vi "Send string wait for return.vi"(0 "VISA resource":refnum<visa-resource-name>, 7 "Command string":string, 9 "Reply expected":bool, 11 "error IO":errorcluster) -> (4 "VISA resource out":refnum<visa-resource-name>, 8 "Reply string":string, 10 "Transmitted":string, 14 "Received Reply":bool, 15 "error out":errorcluster)   [LabVIEW 2011]
doc: "Send a text string to PCP og vent på resultatet om dette er valgt"
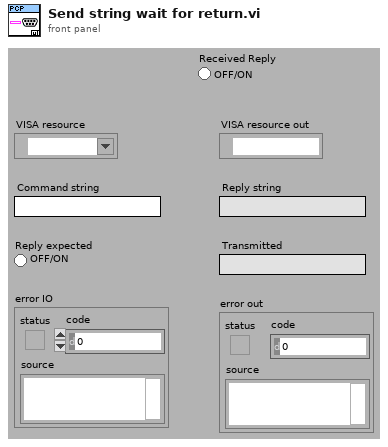
[diagram p1: front panel]
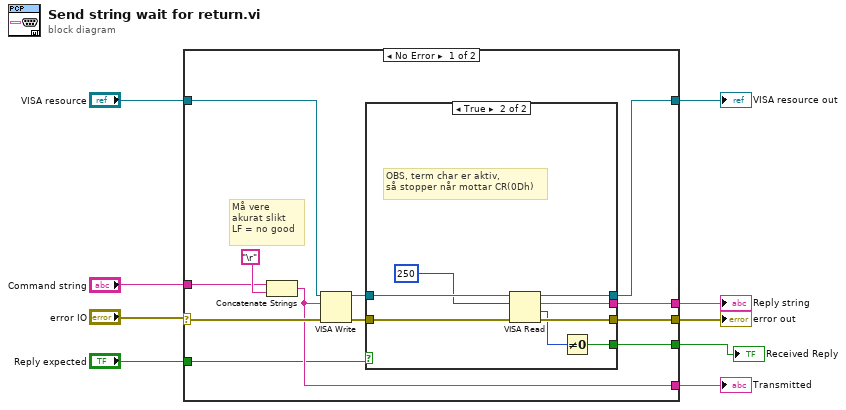
[diagram p0: block diagram]
diagram:
  n1 = case shown="No Error" "error IO" {
    selector: "error IO" -> [w21 w32]
    tunnel: [w17 w33] -> w2
    tunnel: "VISA resource" -> [w20 w33]
    tunnel: [w16 w32] -> w4
    tunnel: [w14 _] -> w5
    tunnel: [w13 _] -> w6
    tunnel: "Command string" -> [w12 _]
    tunnel: "Reply expected" -> [w11 _]
    tunnel: [w10 _] -> w1
    frame No Error {
      # "Må vere \nakurat slikt\nLF = no good"
      n2 = Concatenate Strings(w12, "\r") -> (w14:string)
      n3 = VISA Write(VISA resource name=w20, write buffer=w14, error in (no error)=w21) -> (VISA resource name out=w18:refnum<visa-resource-name>, error out=w19:errorcluster)  [unwired: 1 out]
      n4 = case shown="True" w11 {
        tunnel: w19 -> [w22 w31]
        tunnel: w18 -> [w23 w30]
        tunnel: [w23 w29] -> w17
        tunnel: [w22 w27] -> w16
        tunnel: [_ w26] -> w13
        tunnel: [_ w24] -> w10
        frame False {
          # "Ingen retur forventet"
        }
        frame True {
          # "OBS, term char er aktiv,\nså stopper når mottar CR(0Dh)"
          n5 = VISA Read(VISA resource name=w30, byte count=u32 250 ("Bytes at Port"), error in (no error)=w31) -> (VISA resource name out=w29:refnum<visa-resource-name>, read buffer=w26:string, return count=w25:u32, error out=w27:errorcluster)
          n6 = Not Equal To 0?(x=w25) -> (x != 0?=w24:bool)
        }
      }
    }
    frame Error {
    }
  }
  "Reply string" <- w6
  "Transmitted" <- w5
  "error out" <- w4
  "VISA resource out" <- w2
  "Received Reply" <- w1
